vi "_ReplaceTable.vi"(4 "TableName":string="\"Q1\"", 5 "error in (no error)":errorcluster, 6 "Table":dbl[][](array[numeric])=[[23.0123, 45.0123], [33.0, 55.0]], 7 "ScanModeRefArray":refnum<k20>[](array[refnum]), 8 "DOM Document":refnum<k20>) -> (0 "error out":errorcluster, 2 "ScanModeRefArrayOut":refnum<k20>[](array[refnum]), 3 "DOM DocumentOut":refnum<k20>)   [LabVIEW 2015]
uses:
  <vilib>/xml/Close Reference(Node).vi
  <vilib>/xml/NI_XML.lvlib
  <resource>/objmgr/DOMUserDefRef.rc
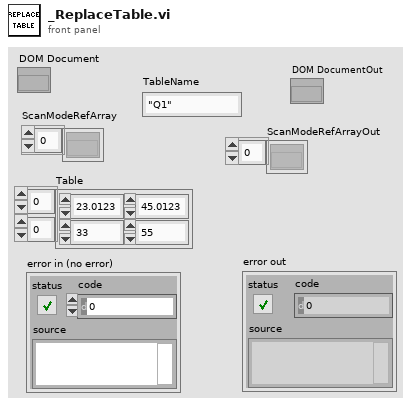
[diagram p1: front panel]
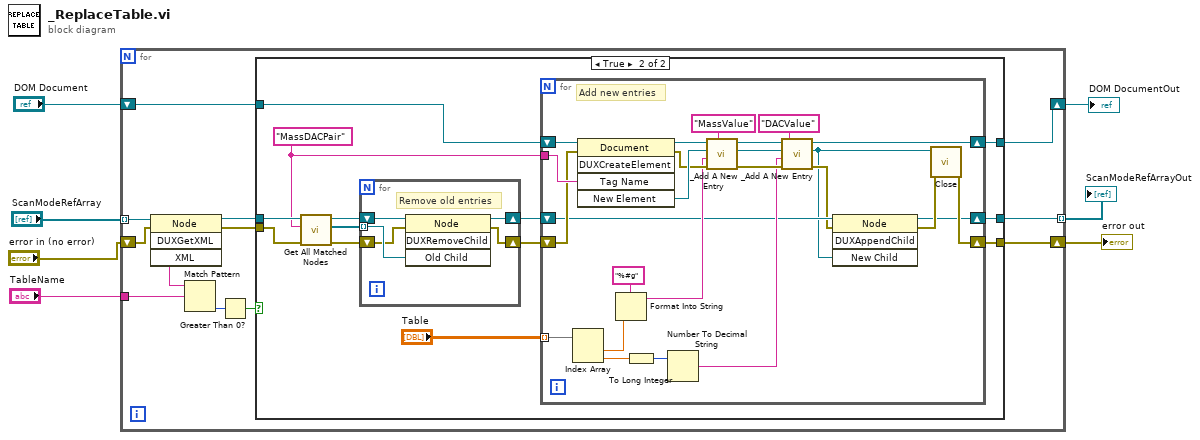
[diagram p0: block diagram]
diagram:
  n1 = for {
    tunnel: "ScanModeRefArray" -> [w18] mode=indexing
    tunnel: "TableName" -> [w15]
    shift-right: [w9] -> w4
    shift-left: "error in (no error)" -> [w19]
    shift-right: [w10] -> w2
    shift-left: "DOM Document" -> [w11]
    tunnel: [w8] -> w1 mode=indexing
    n2 = invoke class="Node" method="DUXGetXML"(reference=w18, error in=w19) -> (reference out=w12:refnum<k20>, error out=w13:errorcluster, "XML"=w16:string)  [unwired: 2 in, 1 out]
    n3 = Match Pattern(string=w16, regular expression=w15) -> (offset past match=w17:i32)  [unwired: 1 in, 3 out]
    n4 = Greater Than 0?(x=w17) -> (x > 0?=w14:bool)
    n5 = case shown="True" w14 {
      tunnel: w13 -> [w22 w34]
      tunnel: [w22 w23] -> w9
      tunnel: w12 -> [w21 w35]
      tunnel: [w21 w26] -> w8
      tunnel: w11 -> [w20 w25]
      tunnel: [w20 w24] -> w10
      frame False {
      }
      frame True {
        w27 = "MassDACPair"
        n6 = call <vilib>:"Get All Matched Nodes.vi"("error in (no error)"=w34, "XPath expression"=w27, "node in"=w35) -> ("error out"=w31:errorcluster, "node result array"=w33:refnum<k20>[], "node out"=w32:refnum<k20>)  [unwired: 6 in]
        n7 = for {
          tunnel: w33 -> [w63] mode=indexing
          shift-right: [w65] -> w30
          shift-left: w31 -> [w61]
          shift-right: [w62] -> w29
          shift-left: w32 -> [w64]
          # "Remove old entries"
          n8 = invoke class="Node" method="DUXRemoveChild"(reference=w64, error in=w61, "Old Child"=w63) -> (reference out=w62:refnum<k20>, error out=w65:errorcluster)  [unwired: 1 in, 2 out]
        }
        n9 = for {
          shift-right: [w38] -> w23
          shift-left: w30 -> [w50]
          shift-right: [w37] -> w26
          shift-left: w29 -> [w42]
          tunnel: "Table" -> [w49] mode=indexing
          tunnel: w27 -> [w59]
          shift-right: [w36] -> w24
          shift-left: w25 -> [w60]
          # "Add new entries"
          n10 = Index Array(array=w49) -> (element #1=w47:dbl, element #2=w46:dbl)  [unwired: 2 in]
          n11 = invoke class="Document" method="DUXCreateElement"(reference=w60, error in=w50, "Tag Name"=w59) -> (reference out=w53:refnum<k20>, error out=w51:errorcluster, "New Element"=w52:refnum<k20>)  [unwired: 2 in, 2 out]
          n12 = Format Into String(format string="%#g", w47) -> (resulting string=w44:string)  [unwired: 2 in, 1 out]
          n13 = To Long Integer(number=w46) -> (32bit integer=w45:i32)
          n14 = Number To Decimal String(number=w45) -> (decimal integer string=w43:string)  [unwired: 1 in]
          n15 = call "_Add A New Entry.vi"("Tag Name"="MassValue", "error in (no error)"=w51, "Data"=w44, "Parent Node"=w52, "DOM document"=w53) -> ("error out"=w55:errorcluster, "Parent Node out"=w54:refnum<k20>, "DOM document out"=w56:refnum<k20>)  [unwired: 1 in]
          n16 = call "_Add A New Entry.vi"("Tag Name"="DACValue", "error in (no error)"=w55, "Data"=w43, "Parent Node"=w54, "DOM document"=w56) -> ("error out"=w41:errorcluster, "Parent Node out"=w40:refnum<k20>, "DOM document out"=w36:refnum<k20>)  [unwired: 1 in]
          n17 = invoke class="Node" method="DUXAppendChild"(reference=w42, error in=w41, "New Child"=w40) -> (reference out=w37:refnum<k20>, error out=w39:errorcluster)  [unwired: 1 in, 2 out]
          n18 = call-poly <vilib>:"Close.vi"("error in (no error)"=w39, "node"=w40) -> ("error out"=w38:errorcluster)  [unwired: 7 in]
        }
      }
    }
  }
  "error out" <- w4
  "DOM DocumentOut" <- w2
  "ScanModeRefArrayOut" <- w1
